vi "Save J-t Data_IIT.vi"(0 "Experiment Indicator":string, 1 "Cell details cluster":T1={"Cell Position"=16, "Cell Label"="", "Pixel to measure"=0, "Area (cm^2)"=0.126, "Variable"="", "Variable value"="", "Scan settings in queue"=0, "Light or dark"=""} {"Pixel to measure" items=["All", "1", "2", "3", "4", "5", "6", "7", "8"]}, 3 "Scan direction":i32, 4 "Data Array":dbl[][](array[numeric]), 6 "Username":string) -> (17 "File path for JV data":path, 18 "File path for JV image":path)   [LabVIEW 2011]
uses:
  <vilib>/Utility/file.llb/Write To Spreadsheet File (string).vi
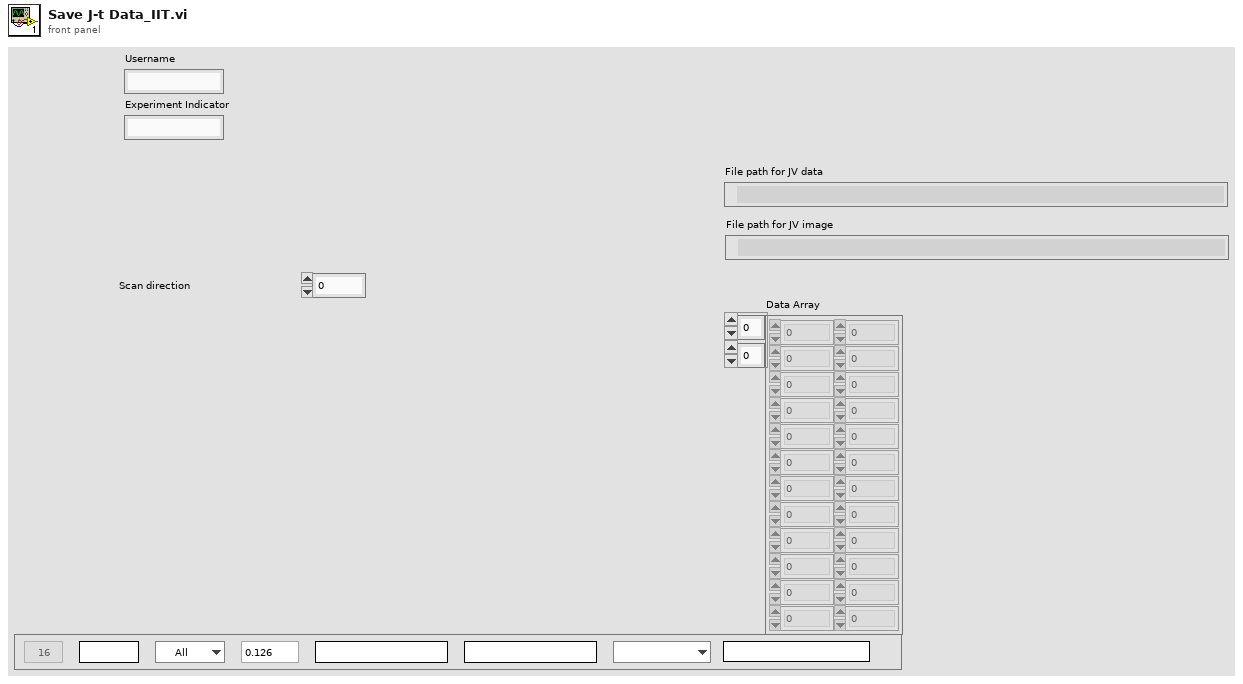
[diagram p1: front panel]
types:
  T1 = cluster{"Cell Position":i32, "Cell Label":string, "Pixel to measure":u16, "Area (cm^2)":dbl, "Variable":string, "Variable value":string, "Scan settings in queue":u16, "Light or dark":string}
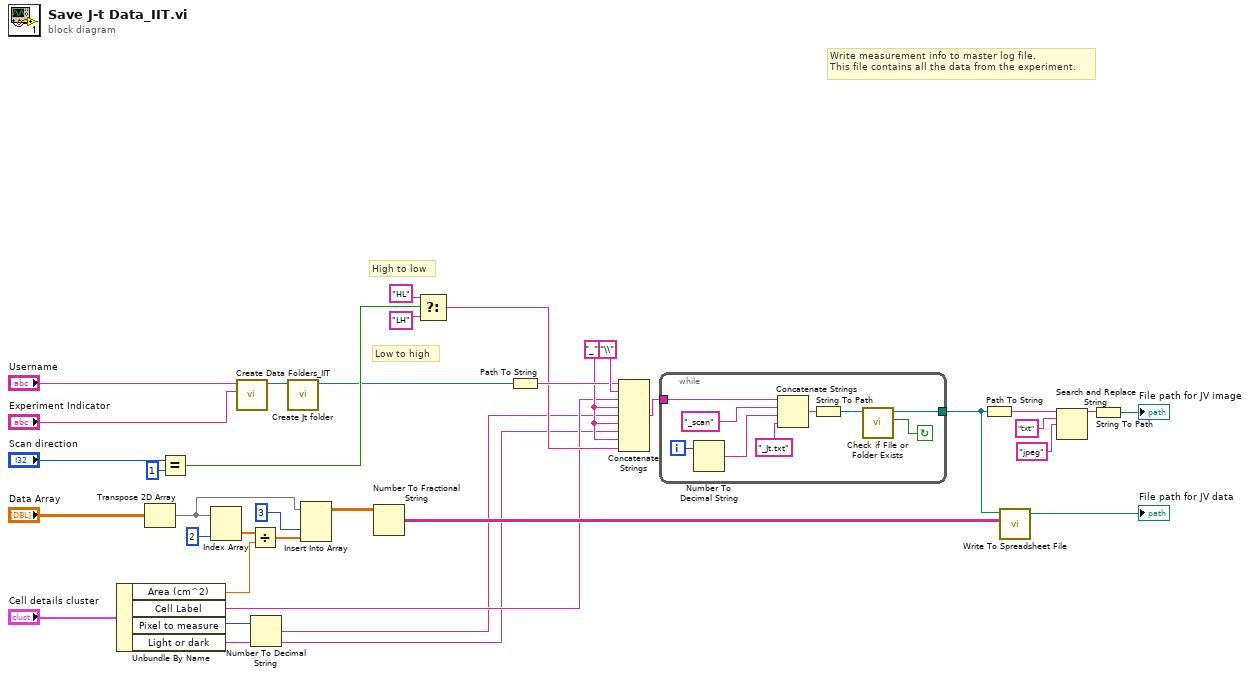
[diagram p0: block diagram]
diagram:
  w18 = "_"
  # "Write measurement info to master log file.\nThis file contains all the data from the experiment."
  # "Low to high"
  # "High to low"
  n1 = Unbundle By Name("Cell details cluster") -> ("Area (cm^2)"=w5:dbl, "Cell Label"=w4:string, "Pixel to measure"=w2:u16, "Light or dark"=w3:string)
  n2 = Transpose 2D Array(2D array="Data Array") -> (transposed array=w11:dbl[][])
  n3 = Equal?(x="Scan direction", y=1) -> (x = y?=w23:bool)
  n4 = Index Array(array=w11, index (col)=2) -> (element=w13:dbl[])  [unwired: 1 in]
  n5 = call "Create Data Folders_IIT.vi"("Experiment Indicator"="Experiment Indicator", "username"="Username") -> ("Data Output Folder"=w8:path)  [unwired: 9 in]
  n6 = Divide(x=w13, y=w5) -> (x/y=w12:dbl[])
  n7 = Number To Decimal String(number=w2) -> (decimal integer string=w1:string)  [unwired: 1 in]
  n8 = call "Create Jt folder.vi"("Data Folder In"=w8) -> ("Data Output Folder"=w7:path)  [unwired: 10 in]
  n9 = Insert Into Array(array=w11, index (col)=3, new element=w12) -> (w9:dbl[][])  [unwired: 1 in]
  n10 = Number To Fractional String(number=w9) -> (F-format string=w15:string[][])  [unwired: 3 in]
  n11 = Select(t="HL", s=w23, f="LH") -> (s? t:f=w17:string)
  n12 = Path To String(path=w7) -> (string=w32:string)
  n13 = Concatenate Strings(w32, "\\", w4, w18, w1, w18, w3, w18, w17) -> (w20:string)
  n14 = while {
    tunnel: w20 -> [w44]
    tunnel: [w36] -> w16
    i -> [w42]
    stop <- w37 continue-if-true
    n15 = Number To Decimal String(number=w42) -> (decimal integer string=w41:string)  [unwired: 1 in]
    n16 = Concatenate Strings(w44, "_scan", w41, "_Jt.txt") -> (w38:string)
    n17 = String To Path(string=w38) -> (path=w39:path)
    n18 = call <vilib>:"Check if File or Folder Exists.vi"("path"=w39) -> ("file or folder exists?"=w37:bool, "dup path"=w36:path)  [unwired: 8 in, 1 out]
  }
  n19 = Path To String(path=w16) -> (string=w19:string)
  n20 = call-poly <vilib>:"Write To Spreadsheet File.vi"("2D data"=w15, "file path (dialog if empty)"=w16) -> ("new file path (Not A Path if cancelled)"=→"File path for JV data":path)  [unwired: 6 in]
  n21 = Search and Replace String(input string=w19, search string="txt", replace string="jpeg") -> (result string=w31:string)  [unwired: 5 in, 3 out]
  n22 = String To Path(string=w31) -> (path=→"File path for JV image":path)
